vi "Initialize-object.vi"(8 "error in (no error)":errorcluster, 10 "VI Reference":refnum<vi>) -> (0 "error out":errorcluster, 3 "Reference out":T1)   [LabVIEW 2013, in "Template-class-by-reference.lvlib" / "Template.lvclass"]
uses:
  Template.lvclass
  Object-reference.ctl
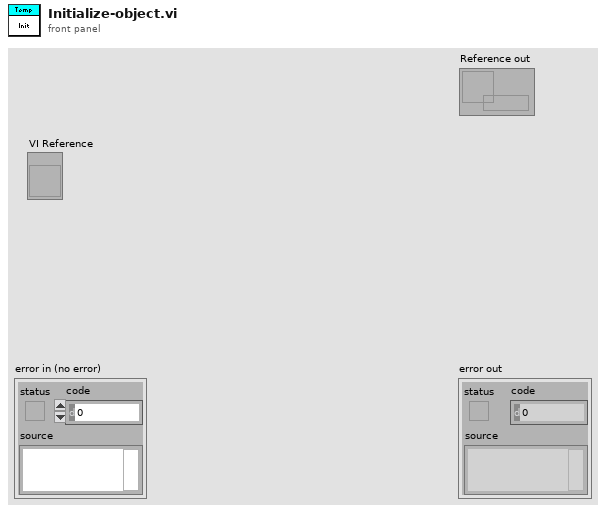
[diagram p1: front panel]
types:
  T1 = typedef "Template-class-by-reference.lvlib/Template.lvclass/Object-reference.ctl" = refnum<data-value>
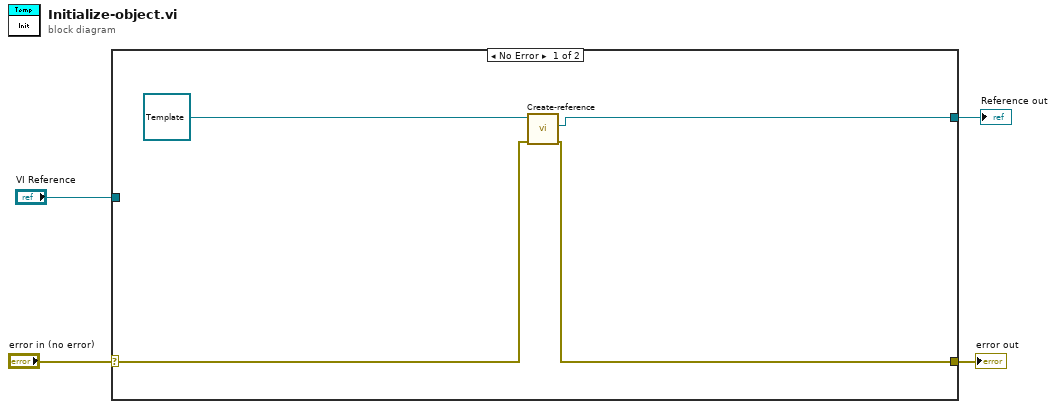
[diagram p0: block diagram]
diagram:
  n1 = case shown="No Error" "error in (no error)" {
    selector: "error in (no error)" -> [w8 w9]
    tunnel: [w6 w9] -> w3
    tunnel: "VI Reference" -> [_ _]
    tunnel: [w5 _] -> w1
    frame No Error {
      n2 = call "Create-reference.vi"("error in (no error)"=w8, "Object in"=refnum<class "Template.lvclass"> refnum ("Panes.lvclass")) -> ("error out"=w6:errorcluster, "Object reference"=w5:T1)  [unwired: 7 in, 1 out]
    }
    frame Error {
    }
  }
  "error out" <- w3
  "Reference out" <- w1
